vi "Get Date String.vi"(8 "error in (no error)":errorcluster, 11 "Type A In":refnum<class "Type A.lvclass">) -> (0 "error out":errorcluster, 2 "Date String":string, 3 "Type A Out":refnum<class "Type A.lvclass">)   [LabVIEW 2020, in "Barcode Reader Second Iteration.lvlib" / "Type A.lvclass"]
uses:
  Type A.lvclass
  Type A.lvclass/Type A.ctl
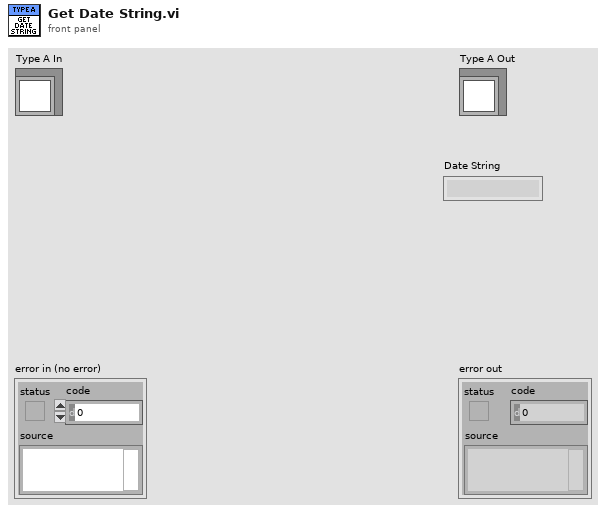
[diagram p1: front panel]
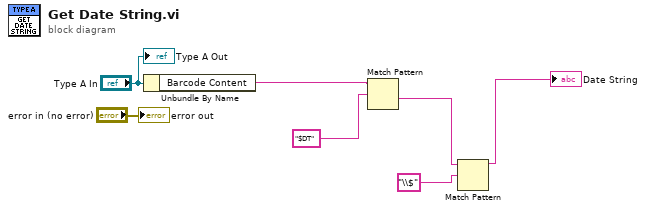
[diagram p0: block diagram]
diagram:
  n1 = Unbundle By Name("Type A In") -> ("Barcode Content"=w5:string)
  n2 = Match Pattern(string=w5, regular expression="$DT" ("format string")) -> (after substring=w3:string)  [unwired: 1 in, 3 out]
  n3 = Match Pattern(string=w3, regular expression="\\$" ("format string")) -> (before substring=→"Date String":string)  [unwired: 1 in, 3 out]
  "error out" <- "error in (no error)"
  "Type A Out" <- "Type A In"
